vi "Dashboard Main.vi"() -> ()   [LabVIEW 2011]
uses:
  KetteringInvitation/Dashboard Datatype.ctl
  <vilib>/Rock Robotics/WPI/DriverStation/WPI_DriverStationDigitalData.ctl
panel:
  in  "Viewer":enum32{"Camera Feed", "Kinect and Info"}(tab)
  out "Camera Image":T1(plugin-control)
  out "Camera Image 2":T1(plugin-control)
  out "Balls in Robot":dbl
  out "Distance":dbl
  out "Shooter Speed":dbl(slide) scale=0.0..1.0
  out "Kinect Calibrate":string
  in  "Harvester":bool=TRUE
  in  "Targets":bool=TRUE
  out "Buttons 1":cluster{"1":bool, "2":bool, "3":bool}
  out "Kinect 1":cluster{"X":dbl, "Y":dbl, "Z":dbl} {"X" scale=1.0..-1.0; "Y" scale=1.0..-1.0; "Z" scale=1.0..-1.0}
  out "Buttons 2":cluster{"1":bool, "2":bool, "3":bool}
  out "Kinect 2":cluster{"X":dbl, "Y":dbl, "Z":dbl} {"X" scale=1.0..-1.0; "Y" scale=1.0..-1.0; "Z" scale=1.0..-1.0}
  out "Version":string
  out "Skeleton Picture":picture
  out "Players":i8
  out "8 -- Battery":sgl(graph)
  out "Analog Input":sgl[](array[slide]) scale=0.0..5.0
  out "PWM":cluster{u8, u8}[](array[slide])=[{0, 157}, {0, 157}, {0, 157}, {0, 157}, {0, 157}, {0, 157}, {0, 157}, {0, 157}, {0, 157}, {0, 169}] scale=1.0..255.0
  out "GPIO Output Enable":bool[](array[boolean])
  out "GPIO State":bool[](array[boolean])
  out "Relay":cluster{"Forward":bool[], "Reverse":bool[]}
  out "Robot IP Address":string
  out "Solenoid Output":bool[](array[boolean])
  out "Dashboard Datatype Warning":string="Warning: The Dashboard Datatype used by the robot project and this dashboard do not match.\nSee diagram for more details."
  out "Image Error Message":string="Timeout in Camera Communications"
  # "Analog #1"
  # "1"
  # "7"
  # "Digital #1"
  # "1"
  # "10"
  # "1"
  # "14"
  # "1"
  # "8"
  # "Communications"
  # "Solenoid #1"
  # "1"
  # "8"
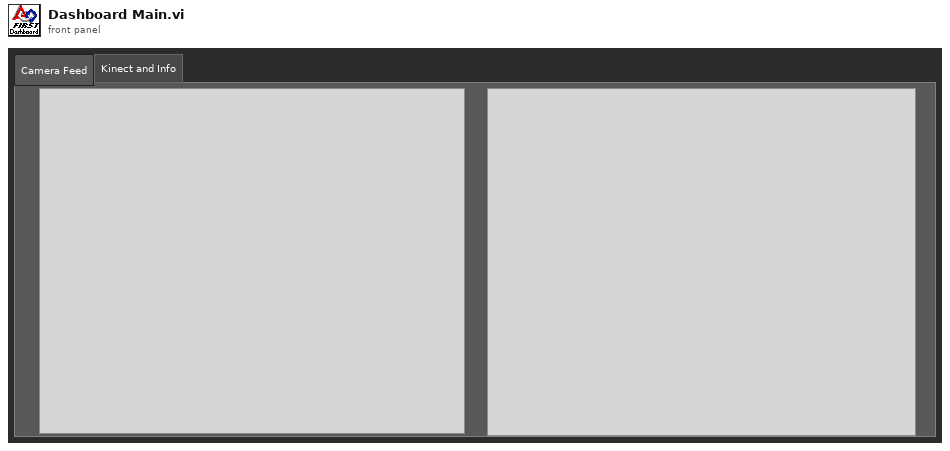
[diagram p1: front panel]
types:
  T1 = typedef "IMAQ Image.ctl" = refnum<image>
  T2 = typedef "Dashboard Datatype.ctl" = cluster{cluster{"AnalogModule[0]":cluster{"Channel[0]":sgl, "Channel[1]":sgl, "Channel[2]":sgl, "Channel[3]":sgl, "Channel[4]":sgl, "Channel[5]":sgl, "Channel[6]":sgl, "Channel[7]":sgl}, "AnalogModule[1]":cluster{"Channel[0]":sgl, "Channel[1]":sgl, "Channel[2]":sgl, "Channel[3]":sgl, "Channel[4]":sgl, "Channel[5]":sgl, "Channel[6]":sgl, "Channel[7]":sgl}}, cluster{"DigitalModule[0]":T3, "DigitalModule[1]":T3}, "Solenoid":u8, "Balls in robot":dbl, "Lock-on":bool, "Shooter Speed":dbl, "Right Drive":dbl, "Left Drive":dbl, "Distance":dbl, "Manual":bool, "Kinect Calibration":string}
  T3 = typedef "WPI_DriverStationDigitalData.ctl" = cluster{"Relay Fwd":u8, "Relay Rev":u8, "GPIO":u16, "GPIO_OE":u16, "PWM":cluster{"PWM[0]":u8, "PWM[1]":u8, "PWM[2]":u8, "PWM[3]":u8, "PWM[4]":u8, "PWM[5]":u8, "PWM[6]":u8, "PWM[7]":u8, "PWM[8]":u8, "PWM[9]":u8}}
  T4 = typedef "Image Type" = u32
  T5 = typedef "LVRectTypeDef.ctl" = cluster{"left":i16, "top":i16, "right":i16, "bottom":i16}
  T6 = cluster{"Competition mode":bool, "Robot Link":bool, "Autonomous":bool, "Enabled":bool, "E-Stop":bool}
  T7 = cluster{"AnalogModule[0]":cluster{"Channel[0]":sgl, "Channel[1]":sgl, "Channel[2]":sgl, "Channel[3]":sgl, "Channel[4]":sgl, "Channel[5]":sgl, "Channel[6]":sgl, "Channel[7]":sgl}, "AnalogModule[1]":cluster{"Channel[0]":sgl, "Channel[1]":sgl, "Channel[2]":sgl, "Channel[3]":sgl, "Channel[4]":sgl, "Channel[5]":sgl, "Channel[6]":sgl, "Channel[7]":sgl}}
  T8 = cluster{"DigitalModule[0]":T3, "DigitalModule[1]":T3}
  T9 = cluster{"Channel[0]":sgl, "Channel[1]":sgl, "Channel[2]":sgl, "Channel[3]":sgl, "Channel[4]":sgl, "Channel[5]":sgl, "Channel[6]":sgl, "Channel[7]":sgl}[]
  T10 = cluster{"Channel[0]":sgl, "Channel[1]":sgl, "Channel[2]":sgl, "Channel[3]":sgl, "Channel[4]":sgl, "Channel[5]":sgl, "Channel[6]":sgl, "Channel[7]":sgl}
  T11 = typedef "SkeletonTrackState.ctl" = enum32{"NotTracked", "PositionOnly", "Tracked"}
  T12 = cluster{"TrackingState":u8[], "Position":cluster{"x":sgl, "y":sgl, "z":sgl}, cluster{"x":sgl, "y":sgl, "z":sgl, sgl}[], "TrackState":T11}
  T13 = cluster{cluster{"ScaledToPercentRange":dbl, "ScaledToPercentRange":dbl, "ScaledToPercentRange":dbl}, cluster{bool, bool, bool}}[]
  T14 = typedef "LVBoundsTypeDef.ctl" = cluster{"Width":u32, "Height":u32}
  T15 = cluster{cluster{"ScaledToPercentRange":dbl, "ScaledToPercentRange":dbl, "ScaledToPercentRange":dbl}, cluster{bool, bool, bool}}
  T16 = cluster{"ScaledToPercentRange":dbl, "ScaledToPercentRange":dbl, "ScaledToPercentRange":dbl}
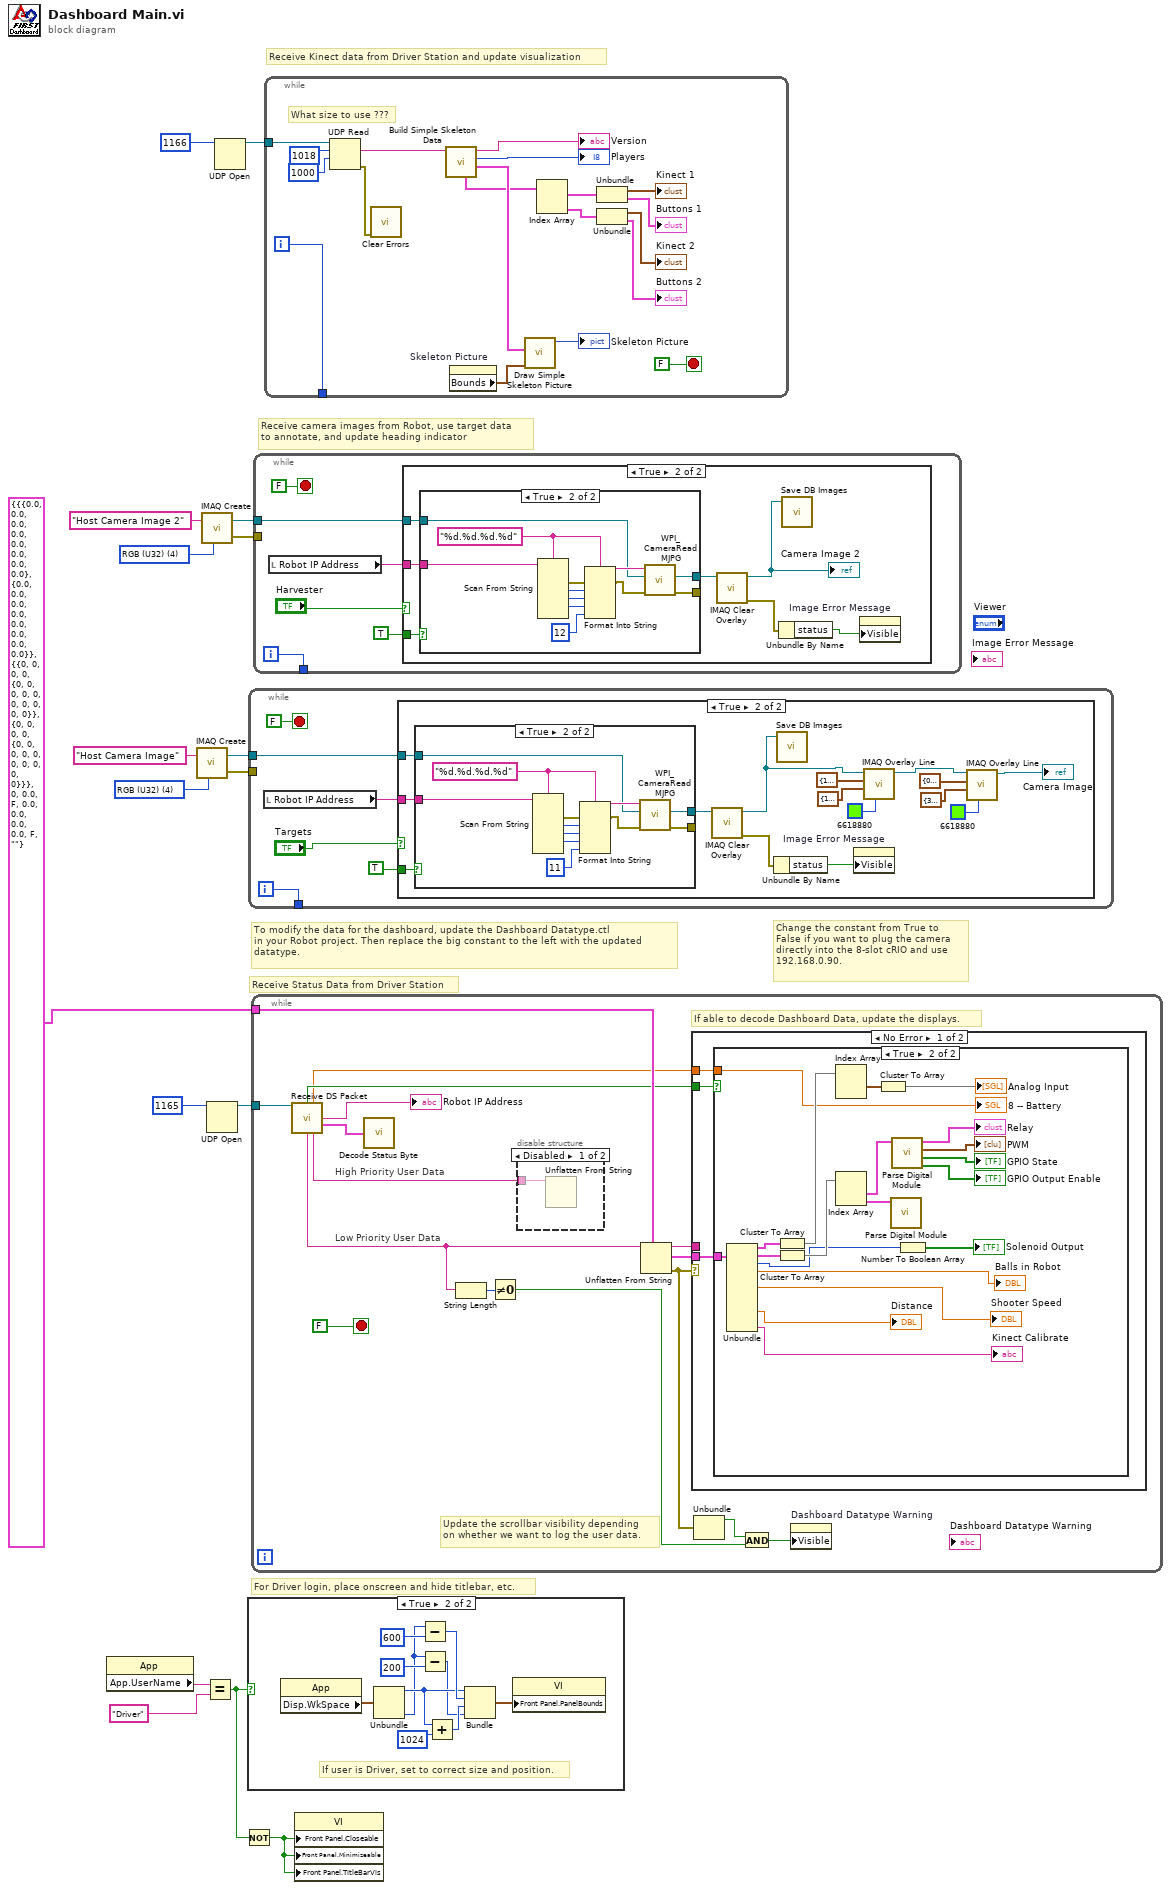
[diagram p0: block diagram]
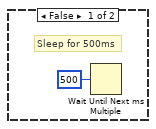
[diagram p2: hidden frame]
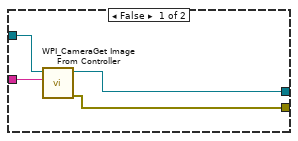
[diagram p3: hidden frame]
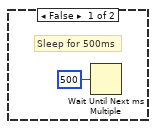
[diagram p8: hidden frame]
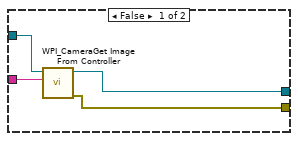
[diagram p9: hidden frame]
diagram:
  w5 = T4 4 items=["Grayscale (U8)", "Grayscale (I16)", "Grayscale (SGL)", "Complex (CSG)", "RGB (U32)", "HSL (U32)", "RGB (U64)"] ("Image Type")
  w15 = T4 4 items=["Grayscale (U8)", "Grayscale (I16)", "Grayscale (SGL)", "Complex (CSG)", "RGB (U32)", "HSL (U32)", "RGB (U64)"] ("Image Type")
  # "Change the constant from True to\nFalse if you want to plug the camera\ndirectly into the 8-slot cRIO and use\n192.168.0.90."
  # "Receive Kinect data from Driver Station and update visualization"
  # "For Driver login, place onscreen and hide titlebar, etc."
  # "To modify the data for the dashboard, update the Dashboard Datatype.ctl\nin your Robot project. Then replace the big constant to the left with the updated\ndatatype."
  # "Receive Status Data from Driver Station"
  # "Receive camera images from Robot, use target data\nto annotate, and update heading indicator"
  n1 = property class="App"() -> ("App.UserName"=w10:string)  [unwired: 2 in, 2 out]
  n2 = call "IMAQ Create"("Image Name"="Host Camera Image", "Image Type"=w15) -> ("New Image"=w13:T1, "error out"=w12:errorcluster)  [unwired: 2 in, 1 out]
  n3 = call "IMAQ Create"("Image Name"="Host Camera Image 2", "Image Type"=w5) -> ("New Image"=w3:T1, "error out"=w2:errorcluster)  [unwired: 2 in, 1 out]
  n4 = Equal?(x=w10, y="Driver") -> (x = y?=w9:bool)
  n5 = UDP Open(11:u16 1165 ("port")) -> (port=w16:refnum<k16>)  [unwired: 2 in, 4 out]
  n6 = UDP Open(11:u16 1166 ("port")) -> (port=w6:refnum<k16>)  [unwired: 2 in, 4 out]
  n7 = Not(x=w9) -> (.not. x?=w8:bool)
  n8 = case shown="True" w9 {
    frame False {
    }
    frame True {
      # "If user is Driver, set to correct size and position."
      n9 = property class="App"() -> ("Disp.WkSpace"=w27:T5)  [unwired: 2 in, 2 out]
      n10 = Unbundle(w27) -> ("left"=w22:i16, "bottom"=w18:i16)  [unwired: 2 out]
      n11 = Subtract(x=w18, y=600) -> (x-y=w24:i32)
      n12 = Subtract(x=w18, y=200) -> (x-y=w19:i32)
      n13 = Add(x=w22, y=1024) -> (x+y=w23:i32)
      n14 = Bundle("left"=w22, w24, w23, w19) -> (w26:cluster{"left":i16, i32, i32, i32})  [unwired: 1 out]
      n15 = property class="VI"("Front Panel.PanelBounds"=w26) -> ()  [unwired: 2 in, 2 out]
    }
  }
  n16 = while {
    tunnel: w13 -> [w31]
    tunnel: w12 -> [_]
    tunnel: [w29] -> _
    i -> [w29]
    stop <- FALSE stop-if-true
    n17 = local read "Robot IP Address"() -> (w32:string)
    n18 = case shown="True" "Targets" {
      tunnel: w32 -> [_ w49]
      tunnel: w31 -> [_ w48]
      tunnel: TRUE -> [_ w44]
      frame False {
        # "Sleep for 500ms"
        n19 = Wait Until Next ms Multiple(millisecond multiple=u32 500) -> ()  [unwired: 1 out]
      }
      frame True {
        n20 = case shown="True" w44 {
          tunnel: w48 -> [w52 w59]
          tunnel: [w50 w57] -> _
          tunnel: [w51 w58] -> w45
          tunnel: w49 -> [w53 w62]
          frame False {
            n21 = call <vilib>:"WPI_CameraGet Image From Controller.vi"("Controller Address"=w53, "Image"=w52) -> ("error out"=w50:errorcluster, "Image Out"=w51:T1)  [unwired: 2 in, 6 out]
          }
          frame True {
            w54 = "%d.%d.%d.%d" ("format string")
            n22 = Scan From String(format string=w54, input string=w62) -> (error out=w61:errorcluster, output 1=w63:i32, output 2=w64:i32, output 3=w65:i32)  [unwired: 2 in, 7 out]
            n23 = Format Into String(format string=w54, error in=w61, w63, w64, w65, 11 ("IP Suffix:")) -> (resulting string=w60:string, error out=w56:errorcluster)  [unwired: 1 in]
            n24 = call <vilib>:"WPI_CameraRead MJPG.vi"("error in"=w56, "Image"=w59, "address"=w60) -> ("error out"=w57:errorcluster, "Image Out"=w58:T1)  [unwired: 7 in]
          }
        }
        n25 = call "IMAQ Clear Overlay"("Image"=w45) -> ("error out"=w46:errorcluster, "Image Out"=w35:T1)  [unwired: 2 in, 7 out]
        n26 = Unbundle By Name(w46) -> ("status"=w47:bool)
        n27 = call "Save DB Images.vi"("Image"=w35) -> ()  [unwired: 2 in, 1 out]
        n28 = property on="Image Error Message" class="Str"("Visible"=w47) -> ()  [unwired: 2 in, 2 out]
        n29 = call "IMAQ Overlay Line"("Color"=u32 6618880, "End Point"=cluster{"X":i32, "Y":i32} {"X"=160, "Y"=240}, "Start Point"=cluster{"X":i32, "Y":i32} {"X"=160, "Y"=0}, "Image"=w35) -> ("Image Out"=w37:T1)  [unwired: 6 in, 1 out]
        n30 = call "IMAQ Overlay Line"("Color"=u32 6618880, "End Point"=cluster{"X":i32, "Y":i32} {"X"=320, "Y"=120}, "Start Point"=cluster{"X":i32, "Y":i32} {"X"=0, "Y"=120}, "Image"=w37) -> ("Image Out"=→"Camera Image":T1)  [unwired: 6 in, 1 out]
      }
    }
  }
  n31 = while {
    tunnel: w16 -> [w79]
    tunnel: T2 {{"AnalogModule[0]"={"Channel[0]"=0.0, "Channel[1]"=0.0, "Channel[2]"=0.0, "Channel[3]"=0.0, "Channel[4]"=0.0, "Channel[5]"=0.0, "Channel[6]"=0.0, "Channel[7]"=0.0}, "AnalogModule[1]"={"Channel[0]"=0.0, "Channel[1]"=0.0, "Channel[2]"=0.0, "Channel[3]"=0.0, "Channel[4]"=0.0, "Channel[5]"=0.0, "Channel[6]"=0.0, "Channel[7]"=0.0}}, {"DigitalModule[0]"={"Relay Fwd"=0, "Relay Rev"=0, "GPIO"=0, "GPIO_OE"=0, "PWM"={"PWM[0]"=0, "PWM[1]"=0, "PWM[2]"=0, "PWM[3]"=0, "PWM[4]"=0, "PWM[5]"=0, "PWM[6]"=0, "PWM[7]"=0, "PWM[8]"=0, "PWM[9]"=0}}, "DigitalModule[1]"={"Relay Fwd"=0, "Relay Rev"=0, "GPIO"=0, "GPIO_OE"=0, "PWM"={"PWM[0]"=0, "PWM[1]"=0, "PWM[2]"=0, "PWM[3]"=0, "PWM[4]"=0, "PWM[5]"=0, "PWM[6]"=0, "PWM[7]"=0, "PWM[8]"=0, "PWM[9]"=0}}}, "Solenoid"=0, "Balls in robot"=0.0, "Lock-on"=FALSE, "Shooter Speed"=0.0, "Right Drive"=0.0, "Left Drive"=0.0, "Distance"=0.0, "Manual"=FALSE, "Kinect Calibration"=""} ("Dashboard Data") -> [w78]
    stop <- FALSE stop-if-true
    # "High Priority User Data"
    # "Low Priority User Data"
    # "Update the scrollbar visibility depending\non whether we want to log the user data."
    # "If able to decode Dashboard Data, update the displays."
    n32 = call "Receive DS Packet.vi"("Recv Socket"=w79) -> ("New Dashboard Data"=w75:bool, "Battery"=w66:sgl, "Robot IP Address"=→"Robot IP Address":string, "Status"=w80:T6, "Low Priority User Data"=w68:string, "High Priority User Data"=w67:string)  [unwired: 1 in, 8 out]
    n33 = call "Decode Status Byte.vi"("Status Byte"=w80) -> ()  [unwired: 2 out]
    n34 = String Length(string=w68) -> (length=w70:i32)
    n35 = Not Equal To 0?(x=w70) -> (x != 0?=w73:bool)
    n36 = disable-structure shown="Disabled" {
      disable-tunnel: w67 -> [w82 _]
      frame Disabled {
        n37 = Unflatten From String(binary string=w82) -> ()  [unwired: 2 in, 5 out]
      }
      frame Enabled {
      }
    }
    n38 = Unflatten From String(type=w78, binary string=w68) -> (rest of the binary string=w71:string, value=w77:T2, error out=w76:errorcluster)  [unwired: 1 in, 2 out]
    n39 = case shown="No Error" w76 {
      tunnel: w77 -> [w85 _]
      tunnel: w75 -> [w84 _]
      tunnel: w71 -> [_ _]
      tunnel: w66 -> [w83 _]
      frame No Error {
        n40 = case shown="True" w84 {
          tunnel: w85 -> [_ w96]
          tunnel: w83 -> [_ w93]
          frame False {
            # "Don't update if the robot hasn't sent new data"
          }
          frame True {
            n41 = Unbundle(w96) -> (w90:T7, w91:T8, "Solenoid"=w92:u8, "Balls in robot"=→"Balls in Robot":dbl, "Shooter Speed"=→"Shooter Speed":dbl, "Distance"=→"Distance":dbl, "Kinect Calibration"=→"Kinect Calibrate":string)  [unwired: 4 out]
            n42 = Cluster To Array(cluster=w90) -> (array=w104:T9)
            n43 = Cluster To Array(cluster=w91) -> (array=w103:T3[])
            n44 = Index Array(array=w104) -> (element #1=w94:T10)  [unwired: 2 in, 1 out]
            n45 = Index Array(array=w103) -> (element #1=w102:T3, element #2=w97:T3)  [unwired: 2 in]
            n46 = Cluster To Array(cluster=w94) -> (array=→"Analog Input":sgl[])
            n47 = call "Parse Digital Module.vi"("DigitalModule"=w97) -> ()  [unwired: 11 out]
            n48 = call "Parse Digital Module.vi"("DigitalModule"=w102) -> ("GPIO Output Enable"=→"GPIO Output Enable":bool[], "GPIO State"=→"GPIO State":bool[], "PWM"=→"PWM":cluster{u8, u8}[], "Relay"=→"Relay":cluster{"Forward":bool[], "Reverse":bool[]})  [unwired: 7 out]
            n49 = Number To Boolean Array(number=w92) -> (Boolean array=→"Solenoid Output":bool[])
            "8 -- Battery" <- w93
          }
        }
      }
      frame Error {
        # "Your datatypes don't match. The Dashboard Datatype.ctl in your Robot project\nand the big constant to the left of the loop need to match."
      }
    }
    n50 = Unbundle(w76) -> ("status"=w72:bool)  [unwired: 2 out]
    n51 = And(x=w72, y=w73) -> (x .and. y?=w74:bool)
    n52 = property on="Dashboard Datatype Warning" class="Str"("Visible"=w74) -> ()  [unwired: 2 in, 2 out]
  }
  n53 = while {
    tunnel: w3 -> [w109]
    tunnel: w2 -> [_]
    tunnel: [w107] -> _
    i -> [w107]
    stop <- FALSE stop-if-true
    n54 = local read "Robot IP Address"() -> (w110:string)
    n55 = case shown="True" "Harvester" {
      tunnel: w110 -> [_ w119]
      tunnel: w109 -> [_ w118]
      tunnel: TRUE -> [_ w115]
      frame False {
        # "Sleep for 500ms"
        n56 = Wait Until Next ms Multiple(millisecond multiple=u32 500) -> ()  [unwired: 1 out]
      }
      frame True {
        n57 = case shown="True" w115 {
          tunnel: w118 -> [w122 w129]
          tunnel: [w120 w127] -> _
          tunnel: [w121 w128] -> w116
          tunnel: w119 -> [w123 w132]
          frame False {
            n58 = call <vilib>:"WPI_CameraGet Image From Controller.vi"("Controller Address"=w123, "Image"=w122) -> ("error out"=w120:errorcluster, "Image Out"=w121:T1)  [unwired: 2 in, 6 out]
          }
          frame True {
            w124 = "%d.%d.%d.%d" ("format string")
            n59 = Scan From String(format string=w124, input string=w132) -> (error out=w131:errorcluster, output 1=w133:i32, output 2=w134:i32, output 3=w135:i32)  [unwired: 2 in, 7 out]
            n60 = Format Into String(format string=w124, error in=w131, w133, w134, w135, 12 ("IP Suffix:")) -> (resulting string=w130:string, error out=w126:errorcluster)  [unwired: 1 in]
            n61 = call <vilib>:"WPI_CameraRead MJPG.vi"("error in"=w126, "Image"=w129, "address"=w130) -> ("error out"=w127:errorcluster, "Image Out"=w128:T1)  [unwired: 7 in]
          }
        }
        n62 = call "IMAQ Clear Overlay"("Image"=w116) -> ("error out"=w117:errorcluster, "Image Out"=w114:T1)  [unwired: 2 in, 7 out]
        "Camera Image 2" <- w114
        n63 = Unbundle By Name(w117) -> ("status"=w113:bool)
        n64 = call "Save DB Images.vi"("Image"=w114) -> ()  [unwired: 2 in, 1 out]
        n65 = property on="Image Error Message" class="Str"("Visible"=w113) -> ()  [unwired: 2 in, 2 out]
      }
    }
  }
  n66 = while {
    tunnel: w6 -> [w152]
    tunnel: [w136] -> _
    i -> [w136]
    stop <- FALSE stop-if-true
    # "What size to use ???"
    n67 = UDP Read(connection ID=w152, max size (548)=1018 ("bytes to read"), timeout ms (25000)=1000) -> (data out=w146:string, error out=w144:errorcluster)  [unwired: 1 in, 3 out]
    n68 = call <vilib>:"Clear Errors.vi"("error in (no error)"=w144) -> ()  [unwired: 6 in, 1 out]
    n69 = call "Build Simple Skeleton Data.vi"("data out"=w146) -> ("Skeleton Data"=w147:T12, "NumPlayers"=→"Players":i8, "Version String"=→"Version":string, "Simple Joystick Info"=w143:T13)  [unwired: 6 in, 1 out]
    n70 = property on="Skeleton Picture" class="Pict"() -> ("Bounds"=w148:T14)  [unwired: 2 in, 2 out]
    n71 = call "Draw Simple Skeleton Picture.vi"("Bounds"=w148, "Simple Skeleton"=w147) -> ("new picture out"=→"Skeleton Picture":picture)  [unwired: 9 in]
    n72 = Index Array(array=w143) -> (element #1=w142:T15, element #2=w141:T15)  [unwired: 2 in]
    n73 = Unbundle(w142) -> (→"Kinect 1":T16, →"Buttons 1":cluster{bool, bool, bool})
    n74 = Unbundle(w141) -> (→"Kinect 2":T16, →"Buttons 2":cluster{bool, bool, bool})
  }
  n75 = property class="VI"("Front Panel.Closeable"=w8, "Front Panel.Minimizeable"=w8, "Front Panel.TitleBarVis"=w8) -> ()  [unwired: 2 in, 2 out]
